vi "create_s3.vi"(10 "Path":string) -> (3 "source":refnum<class "s3.lvclass">)   [LabVIEW 2020, in "datasources.lvlib" / "source.lvclass"]
uses:
  source.lvclass
  s3/s3.lvclass
  C:/code/labview-client/lv_src/Nominal Client/datasources/source/source.lvclass
  source.lvclass/source.ctl
  path.set.vi
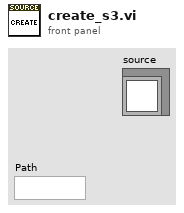
[diagram p1: front panel]
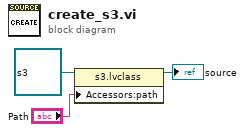
[diagram p0: block diagram]
diagram:
  n1 = property class="s3.lvclass"(reference=refnum<class "s3.lvclass"> refnum ("datasources.lvlib:s3.lvclass"), "Accessors:path"="Path") -> (reference out=→"source":refnum<class "s3.lvclass">)  [unwired: 1 in, 1 out]
